vi "add.vi"(8 "error in (no error)":errorcluster, 9 "addend":dbl, 10 "addend":refnum<class "ImageCollection.lvclass">, 11 "ImageCollection in":refnum<class "ImageCollection.lvclass">) -> (0 "error out":errorcluster, 3 "ImageCollection out":refnum<class "ImageCollection.lvclass">)   [LabVIEW 2010, in "ImageCollection.lvclass"]
uses:
  ImageCollection.lvclass
  Image/Image/Image.lvclass
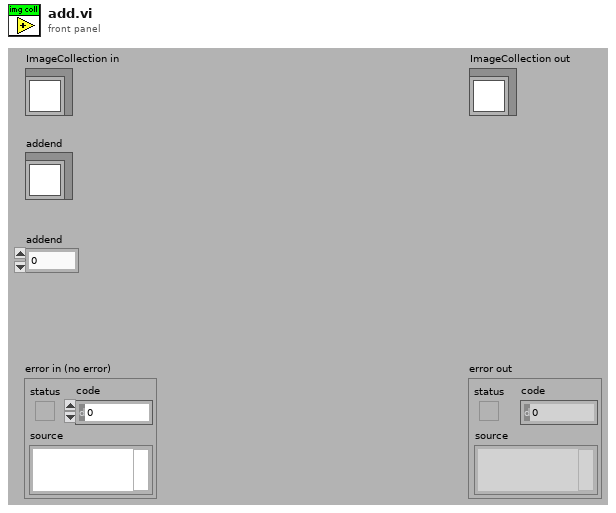
[diagram p1: front panel]
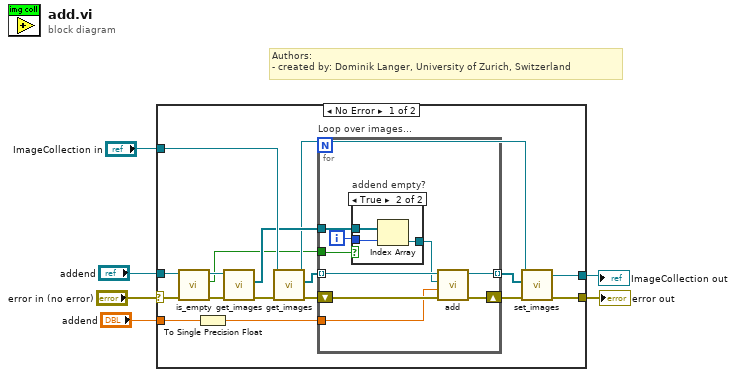
[diagram p0: block diagram]
diagram:
  # "Authors: \n- created by: Dominik Langer, University of Zurich, Switzerland"
  n1 = case shown="No Error" "error in (no error)" {
    selector: "error in (no error)" -> [w9 w37]
    tunnel: [w16 w37] -> w5
    tunnel: [w14 w36] -> w6
    tunnel: "ImageCollection in" -> [w23 w36]
    tunnel: "addend" -> [w12 _]
    tunnel: "addend" -> [w13 _]
    frame No Error {
      n2 = call "is_empty.vi"("error in (no error)"=w9, "ImageCollection in"=w12) -> ("error out"=w10:errorcluster, "is empty?"=w8:bool, "ImageCollection out"=w11:refnum<class "ImageCollection.lvclass">)  [unwired: 7 in]
      n3 = To Single Precision Float(number=w13) -> (single precision float=w7:sgl)
      n4 = call-dynamic "get_images.vi"("error in (no error)"=w10, "ImageCollection.lvclass in"=w11) -> ("error out"=w20:errorcluster, "images"=w19:refnum<class "Image.lvclass">[])  [unwired: 8 out]
      n5 = call-dynamic "get_images.vi"("error in (no error)"=w20, "ImageCollection.lvclass in"=w23) -> ("error out"=w22:errorcluster, "images"=w21:refnum<class "Image.lvclass">[], "ImageCollection.lvclass out"=w15:refnum<class "ImageCollection.lvclass">)  [unwired: 7 out]
      n6 = for "Loop over images..." {
        tunnel: w21 -> [w31] mode=indexing
        tunnel: w19 -> [w27]
        shift-right: [w30] -> w18
        shift-left: w22 -> [w32]
        tunnel: [w29] -> w17 mode=indexing
        tunnel: w7 -> [w28]
        tunnel: w8 -> [w25]
        i -> [w26]
        n7 = case "addend empty?" shown="True" w25 {
          tunnel: w27 -> [_ w35]
          tunnel: w26 -> [_ w34]
          tunnel: [_ w33] -> w24
          frame False {
          }
          frame True {
            n8 = Index Array(array=w35, index=w34) -> (element=w33:refnum<class "Image.lvclass">)
          }
        }
        n9 = call-dynamic "add.vi"("error in (no error)"=w32, "constant"=w28, "addend"=w24, "Image in"=w31) -> ("error out"=w30:errorcluster, "Image out"=w29:refnum<class "Image.lvclass">)  [unwired: 6 out]
      }
      n10 = call-dynamic "set_images.vi"("error in (no error)"=w18, "images"=w17, "ImageCollection.lvclass in"=w15) -> ("error out"=w16:errorcluster, "ImageCollection.lvclass out"=w14:refnum<class "ImageCollection.lvclass">)  [unwired: 7 out]
    }
    frame Error {
    }
  }
  "error out" <- w5
  "ImageCollection out" <- w6
